vi "Count Down U8.vi"(9 "reset value":u8, 10 "reset":bool, 11 "decrement":bool) -> (3 "count":u8)   [LabVIEW 2013, in "I2S-TDM.lvlib"]
uses:
  I2S-TDM.lvlib
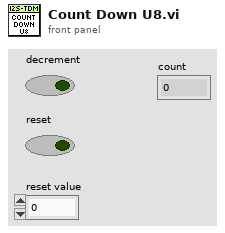
[diagram p1: front panel]
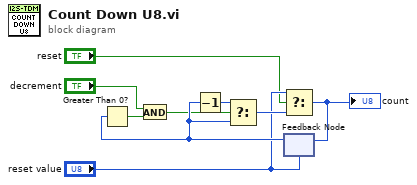
[diagram p0: block diagram]
diagram:
  n1 = feedback #1("reset value") -> (w8:u8)
  n2 = Greater Than 0?(x=w8) -> (x > 0?=w7:bool)
  n3 = And(x="decrement", y=w7) -> (x .and. y?=w5:bool)
  n4 = Decrement(x=w8) -> (x-1=w9:u8)
  n5 = Select(t=w9, s=w5, f=w8) -> (s? t:f=w4:u8)
  n6 = Select(t="reset value", s="reset", f=w4) -> (s? t:f=w1:u8)
  "count" <- w1
  n7 = feedback-in #1(w1) -> ()
